vi "Math Eval y=f(x).vi"(6 "formula":string, 8 "Error In":errorcluster, 9 "start":dbl format="%.2f", 10 "end":dbl=1.0 format="%.2f", 11 "number of points":u32=10) -> (0 "Error Out":errorcluster, 2 "Y Values":dbl[](array[numeric]) format="%.2f", 3 "X Values":dbl[](array[numeric]) format="%.2f", 4 "CPU (s)":dbl)   [LabVIEW 2021, in "Math.lvlib"]
uses:
  <vilib>/Utility/error.llb/Error Cluster From Error Code.vi
  <vilib>/ErrorRing/Error Ring.xnode
  Math.lvlib
  <vilib>/gmath/NI_Gmath.lvlib
  Time/Time.lvlib
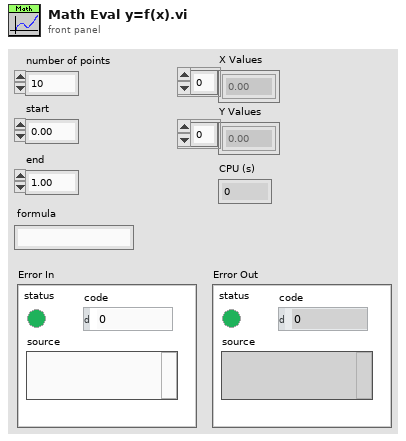
[diagram p1: front panel]
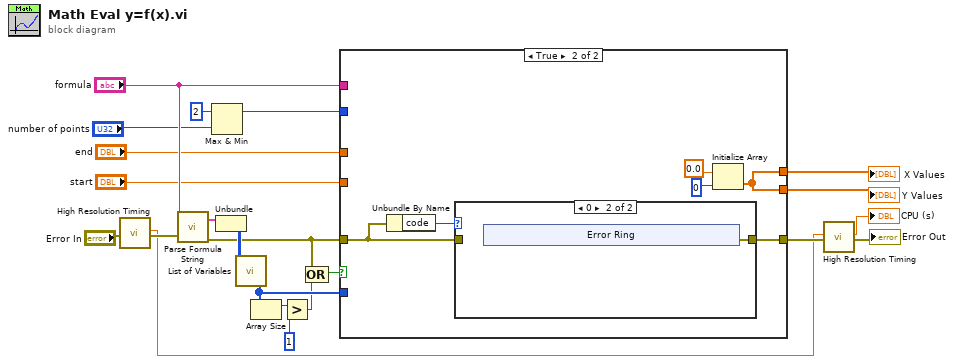
[diagram p0: block diagram]
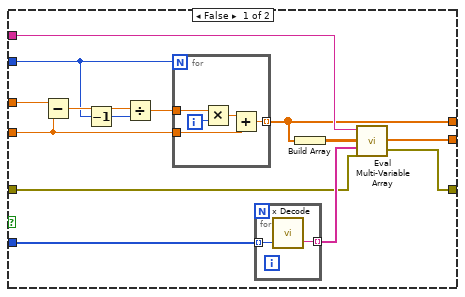
[diagram p2: hidden frame]
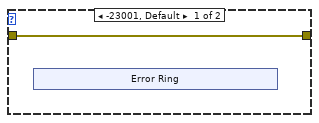
[diagram p3: hidden frame]
diagram:
  n1 = call "High Resolution Timing.vi"("Error In"="Error In") -> ("elapsed (relative) seconds"=w5:dbl, "Error Out"=w8:errorcluster)  [unwired: 16 in, 1 out]
  n2 = call <vilib>:"Parse Formula String.vi"("error in (no error)"=w8, "formula"="formula") -> ("error out"=w3:errorcluster, "Parsed Formula"=w15:cluster{"Table":i32[][], "Y Values":dbl[]})
  n3 = Max & Min(x=u32 2, y="number of points") -> (max(x,y)=w1:u32)  [unwired: 1 out]
  n4 = Unbundle(w15) -> ("Table"=w14:i32[][])  [unwired: 1 out]
  n5 = call <vilib>:"List of Variables.vi"("Table"=w14) -> ("List of variables"=w19:i32[])
  n6 = Array Size(array=w19) -> (size(s)=w21:i32)
  n7 = Greater?(x=w21, y=1) -> (0:w16:bool)
  n8 = Compound Arithmetic op=OR(w3, w16) -> (w22:bool)
  n9 = case shown="True" w22 {
    tunnel: "formula" -> [w36 _]
    tunnel: w19 -> [w35 _]
    tunnel: [w31 w44] -> w18
    tunnel: [w34 w44] -> w17
    tunnel: w1 -> [w28 _]
    tunnel: "end" -> [w27 _]
    tunnel: "start" -> [w26 _]
    tunnel: [w24 w46] -> w7
    tunnel: w3 -> [w23 w45]
    frame False {
      n10 = Subtract(x=w27, y=w26) -> (x-y=w32:dbl)
      n11 = Decrement(x=w28) -> (x-1=w25:u32)
      n12 = Divide(x=w32, y=w25) -> (x/y=w33:dbl)
      n13 = for {
        N: w28 -> [_]
        tunnel: w33 -> [w43]
        tunnel: w26 -> [w40]
        tunnel: [w39] -> w31 mode=indexing
        i -> [w42]
        n14 = Multiply(x=w43, y=w42) -> (x*y=w41:dbl)
        n15 = Add(x=w41, y=w40) -> (x+y=w39:dbl)
      }
      n16 = for {
        tunnel: w35 -> [w38] mode=indexing
        tunnel: [w37] -> w29 mode=indexing
        n17 = call <vilib>:"x Decode.vi"("number"=w38) -> ("x string"=w37:string)  [unwired: 1 in, 1 out]
      }
      n18 = Build Array(w31) -> (w30:dbl[][])
      n19 = call <vilib>:"Eval Multi-Variable Array.vi"("error in (no error)"=w23, "Variables"=w29, "X Values"=w30, "formula"=w36) -> ("error out"=w24:errorcluster, "Y Values"=w34:dbl[])
    }
    frame True {
      n20 = Unbundle By Name(w45) -> ("code"=w47:i32)
      n21 = case shown="0" w47 {
        tunnel: [w50 w55] -> w46
        tunnel: w45 -> [w50 _]
        frame -23001, Default {
          n22 = xnode "Error Ring"() -> ()  [unwired: 1 out]
        }
        frame 0 {
          n23 = xnode "Error Ring"() -> ("error out"=w55:errorcluster)
        }
      }
      n24 = Initialize Array(0.0, 0) -> (w44:dbl[])
    }
  }
  "X Values" <- w18
  "Y Values" <- w17
  n25 = call "High Resolution Timing.vi"("relative seconds (NaN)"=w5, "Error In"=w7) -> ("elapsed (relative) seconds"=→"CPU (s)":dbl, "Error Out"=→"Error Out":errorcluster)  [unwired: 15 in, 1 out]
